vi "Extract Steps.vi"(1 "Instructions":string="10R5L5R10L4R5L5") -> (0 "Steps":T1[](array[typedef]))   [LabVIEW 2020, in "AoC 2022.lvlib"]
uses:
  AoC 2022.lvlib
  Map Action.ctl
  Map Direction.ctl
  Map Action Step.ctl
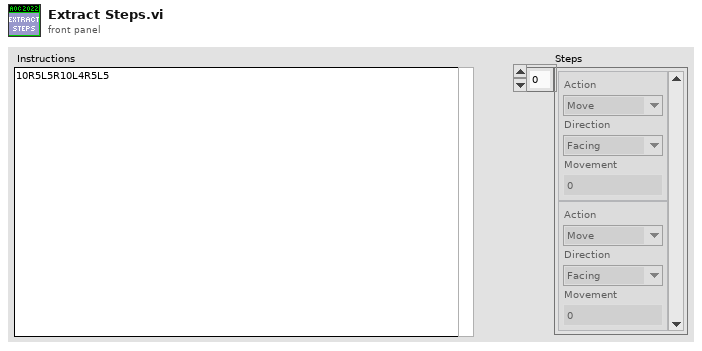
[diagram p1: front panel]
types:
  T1 = typedef "AoC 2022.lvlib/Map Action Step.ctl" = cluster{"Action":T2, "Direction":T3, "Movement":i32}
  T2 = typedef "AoC 2022.lvlib/Map Action.ctl" = enum16{"Move", "Turn"}
  T3 = typedef "AoC 2022.lvlib/Map Direction.ctl" = enum16{"Facing", "Right", "Left", "Up", "Down"}
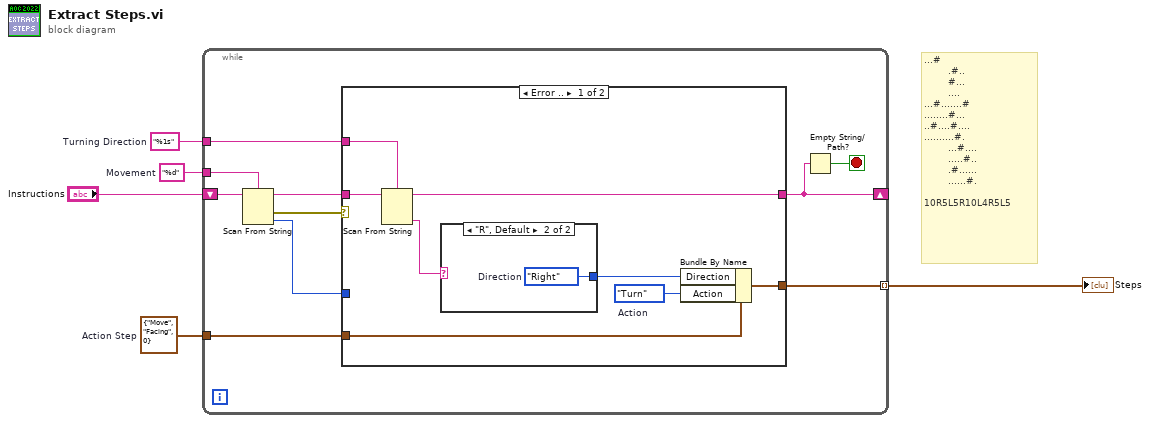
[diagram p0: block diagram]
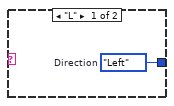
[diagram p2: hidden frame]
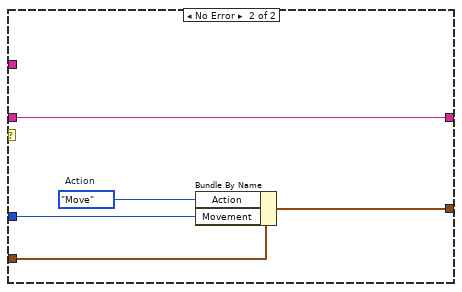
[diagram p3: hidden frame]
diagram:
  w2 = T1 {"Action"=enum."Move", "Direction"=enum."Facing", "Movement"=0}  # Action Step
  w5 = "%d"  # Movement
  w4 = "%1s"  # Turning Direction
  # "...#\n        .#..\n        #...\n        ....\n...#.......#\n........#...\n..#....#....\n..........#.\n        ...#....\n        .....#..\n        .#......\n        ......#.\n\n10R5L5R10L4R5L5"
  n1 = while {
    shift-right: [w14] -> _
    shift-left: "Instructions" -> [w11]
    tunnel: w2 -> [w13]
    tunnel: [w12] -> w3 mode=indexing
    tunnel: w4 -> [w9]
    tunnel: w5 -> [w8]
    stop <- w15 stop-if-true
    n2 = Scan From String(format string=w8, input string=w11) -> (remaining string=w10:string, error out=w6:errorcluster, output 1=w7:i32)  [unwired: 3 in, 1 out]
    n3 = case shown="Error .." w6 {
      tunnel: w10 -> [w20 w30]
      tunnel: [w19 w30] -> w14
      tunnel: w13 -> [w23 w29]
      tunnel: [w21 w27] -> w12
      tunnel: w9 -> [w16 _]
      tunnel: w7 -> [_ w26]
      frame Error {
        w22 = Map_Action."Turn"  # Action
        n4 = Scan From String(format string=w16, input string=w20) -> (remaining string=w19:string, output 1=w18:string)  [unwired: 3 in, 2 out]
        n5 = case shown="\"R\", Default" w18 {
          tunnel: [w24 w25] -> w17
          frame "L" {
            w24 = Map_Direction."Left"  # Direction
          }
          frame "R", Default {
            w25 = Map_Direction."Right"  # Direction
          }
        }
        n6 = Bundle By Name(cluster=w23, "Direction"=w17, "Action"=w22) -> (w21:T1)
      }
      frame No Error {
        w28 = Map_Action."Move"  # Action
        n7 = Bundle By Name(cluster=w29, "Action"=w28, "Movement"=w26) -> (w27:T1)
      }
    }
    n8 = Empty String/Path?(string/path=w14) -> (empty?=w15:bool)
  }
  "Steps" <- w3
